vi "Configure List.vi"(6 "List Step  (1: Auto)":i32(ring)=1 items=["Once", "Auto"], 7 "Last Termination (F: Off)":bool, 8 "error in (no error)":errorcluster {"code" format="%.0x"}, 9 "List Count (1)":i32=1, 10 "Channel Name (1)":string="1", 11 "VISA resource name":refnum<visa-resource-name>) -> (0 "error out":errorcluster {"code" format="%.0x"}, 3 "VISA resource name out":refnum<visa-resource-name>)   [LabVIEW 2016, in "Agilent N6700 Series.lvlib"]
doc: "Configures list properties.\n\n<b>Note:</b>\nThis VI only applies to models N676xA, N678xA SMU, or models that have Option 054 (High-Speed Test Extensions)."
uses:
  <instrlib>/Agilent N6700 Series/Agilent N6700 Series.lvlib
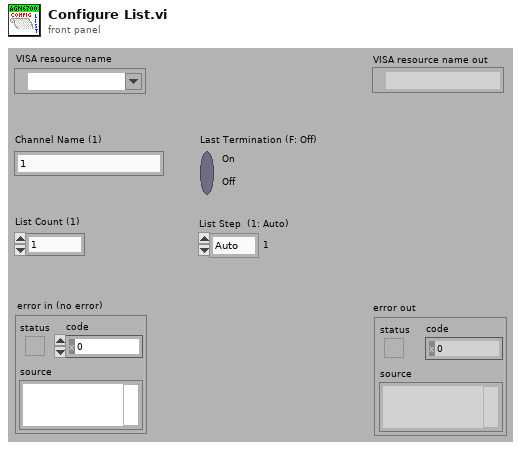
[diagram p1: front panel]
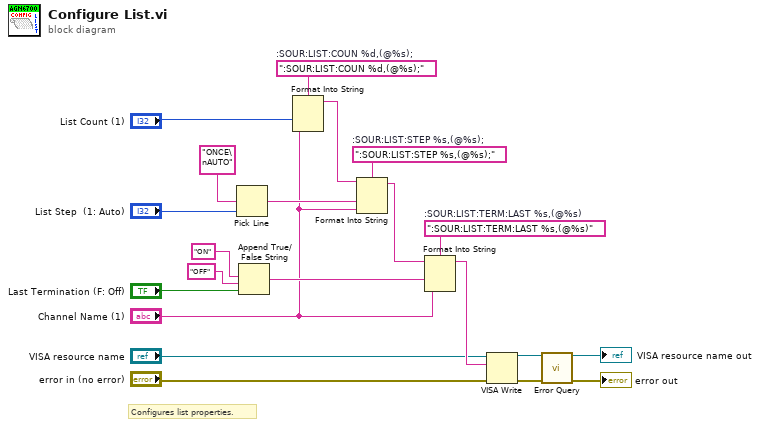
[diagram p0: block diagram]
diagram:
  w9 = ":SOUR:LIST:COUN %d,(@%s);"  # :SOUR:LIST:COUN %d,(@%s);
  w10 = ":SOUR:LIST:STEP %s,(@%s);"  # :SOUR:LIST:STEP %s,(@%s);
  w21 = ":SOUR:LIST:TERM:LAST %s,(@%s)"  # :SOUR:LIST:TERM:LAST %s,(@%s)
  # "Configures list properties."
  n1 = Pick Line(multi-line string="ONCE\nAUTO", line index="List Step  (1: Auto)") -> (output string=w17:string)  [unwired: 1 in]
  n2 = Append True/False String(1:"Last Termination (F: Off)", 2:"OFF", 3:"ON") -> (0:w12:string)  [unwired: 1 in]
  n3 = Format Into String(format string=w9, "List Count (1)", "Channel Name (1)") -> (resulting string=w6:string)  [unwired: 2 in, 1 out]
  n4 = Format Into String(format string=w10, initial string=w6, w17, "Channel Name (1)") -> (resulting string=w5:string)  [unwired: 1 in, 1 out]
  n5 = Format Into String(format string=w21, initial string=w5, w12, "Channel Name (1)") -> (resulting string=w20:string)  [unwired: 1 in, 1 out]
  n6 = VISA Write(VISA resource name="VISA resource name", write buffer=w20, error in (no error)="error in (no error)") -> (VISA resource name out=w2:refnum<visa-resource-name>, error out=w1:errorcluster)  [unwired: 1 out]
  n7 = call <instrlib>:"Error Query.vi"("VISA resource name"=w2, "error in (no error)"=w1) -> ("VISA resource name out"=→"VISA resource name out":refnum<visa-resource-name>, "error out"=→"error out":errorcluster)  [unwired: 10 in, 2 out]
